vi "Send Control Message.vi"(8 "error in (no error)":errorcluster, 10 "Message":string, 11 "Sift Client in":refnum<class "Sift Client.lvclass">) -> (0 "error out":errorcluster, 3 "Sift Client out":refnum<class "Sift Client.lvclass">)   [LabVIEW 2024, in "Sift Client.lvlib" / "Sift Client.lvclass"]
uses:
  Sift Client.lvclass
  Sift Client.lvclass/Sift Client.ctl
  Sift Client.lvlib
panel:
  out "Response":string
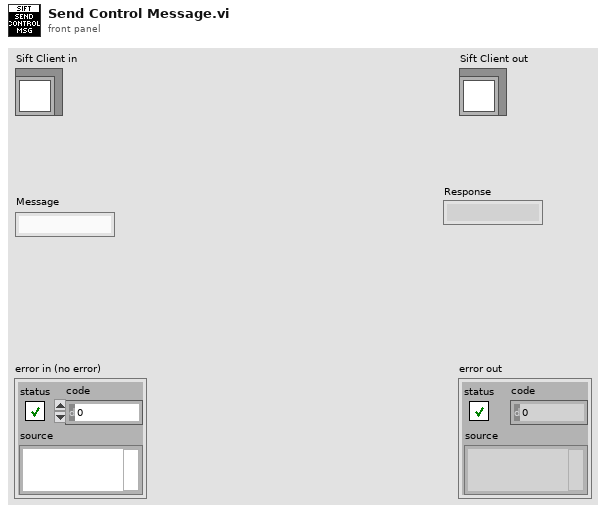
[diagram p1: front panel]
types:
  T1 = enum16{"Standard", "Buffered", "CRLF", "Immediate"}
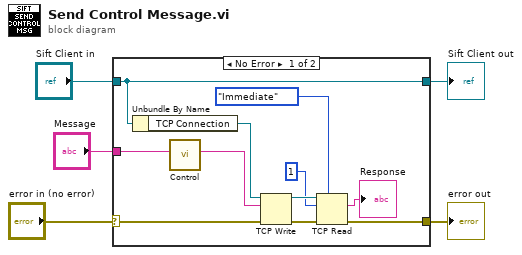
[diagram p0: block diagram]
diagram:
  n1 = case shown="No Error" "error in (no error)" {
    selector: "error in (no error)" -> [w13 w18]
    tunnel: [w7 w18] -> w4
    tunnel: [w15 w17] -> w2
    tunnel: "Sift Client in" -> [w15 w17]
    tunnel: "Message" -> [w12 _]
    frame No Error {
      n2 = Unbundle By Name(w15) -> ("TCP Connection"=w14:refnum<k5>)
      n3 = call "Control.vi"("Data"=w12) -> ("Message"=w16:string)  [unwired: 10 in]
      n4 = TCP Write(connection ID=w14, data in=w16, error in (no error)=w13) -> (connection ID out=w11:refnum<k5>, error out=w8:errorcluster)  [unwired: 1 in, 1 out]
      n5 = TCP Read(connection ID=w11, bytes to read=1, error in (no error)=w8, 7:T1."Immediate" ("mode (standard)")) -> (data out=→"Response":string, error out=w7:errorcluster)  [unwired: 1 in, 1 out]
    }
    frame Error {
    }
  }
  "error out" <- w4
  "Sift Client out" <- w2
